vi "NI MAX DAY 2 (11.03.2025) (1).vi"() -> ()   [LabVIEW 2025]
panel:
  out "Boolean 2":bool
  in  "stop 2":bool
  in  "stop":bool
  out "Boolean":bool
  out "Numeric 2":i32
  out "Numeric":i32
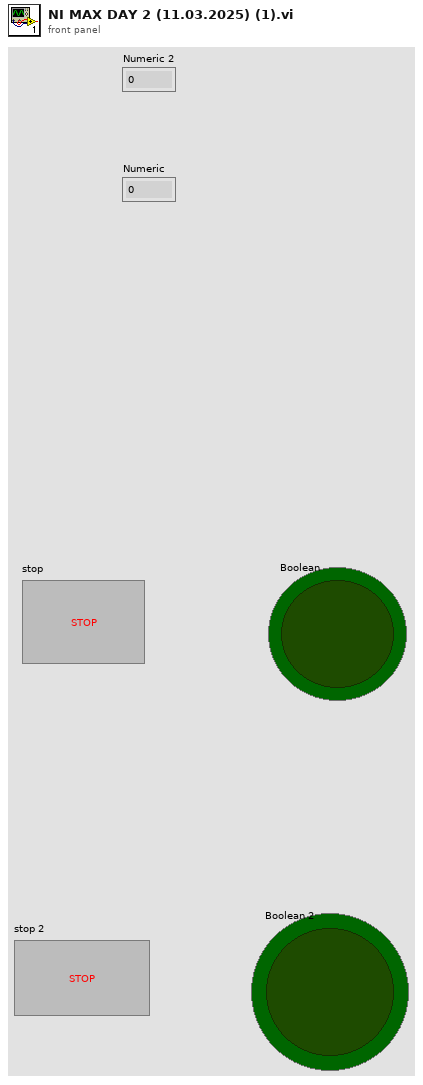
[diagram p1: front panel]
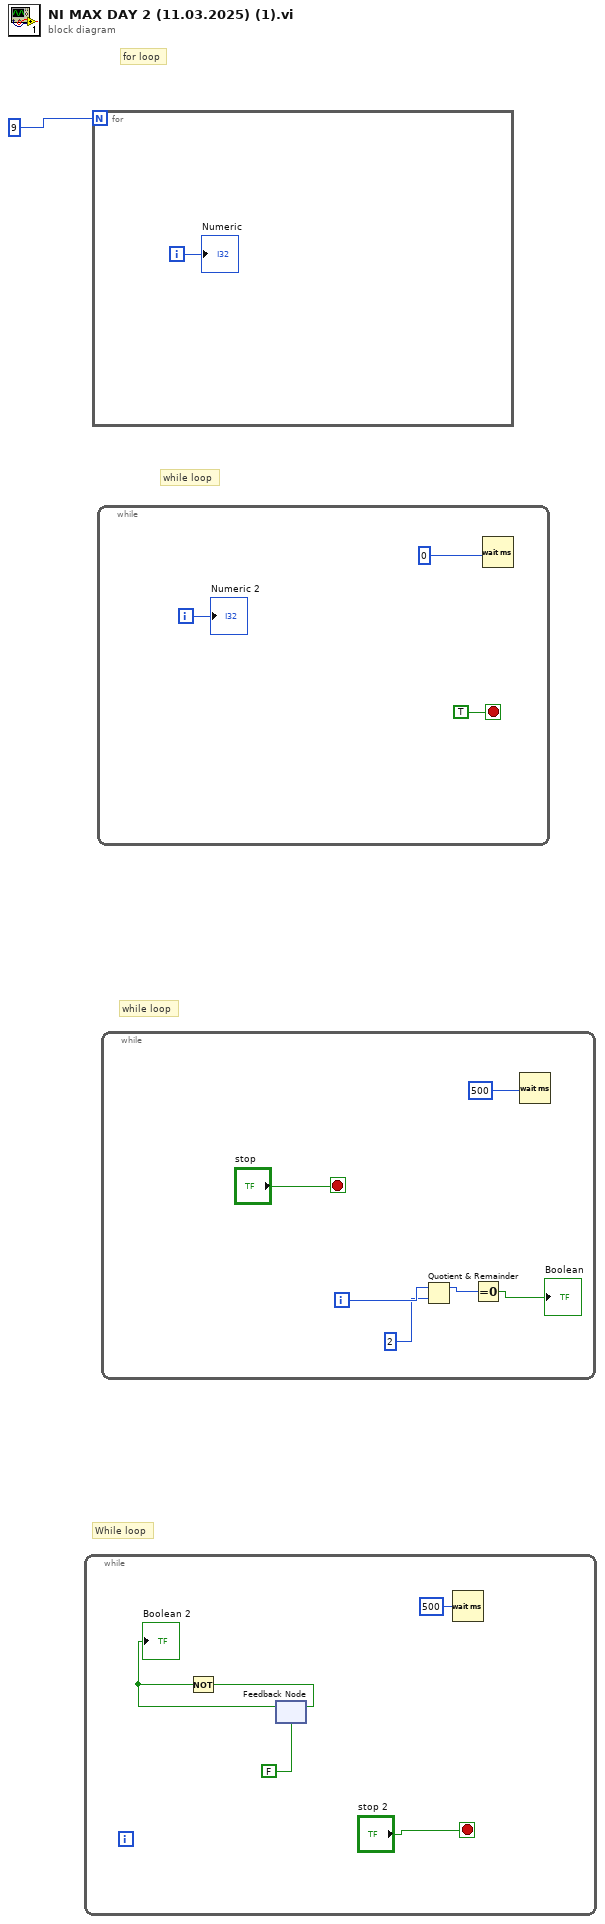
[diagram p0: block diagram]
diagram:
  # "While loop"
  # "for loop"
  # "while loop"
  # "while loop"
  n1 = while {
    stop <- "stop 2" stop-if-true
    n2 = feedback #1(FALSE) -> (w3:bool)
    "Boolean 2" <- w3
    n3 = Not(x=w3) -> (.not. x?=w2:bool)
    n4 = feedback-in #1(w2) -> ()
    n5 = Wait (ms)(milliseconds to wait=u32 500) -> ()  [unwired: 1 out]
  }
  n6 = for {
    N: 9 -> [_]
    i -> [w7]
    "Numeric" <- w7
  }
  n7 = while {
    i -> [w10]
    stop <- TRUE stop-if-true
    n8 = Wait (ms)(milliseconds to wait=u32 0 ("millisecond timer value")) -> ()  [unwired: 1 out]
    "Numeric 2" <- w10
  }
  n9 = while {
    i -> [w14]
    stop <- "stop" stop-if-true
    n10 = Quotient & Remainder(x=w14, y=2 ("floor(x/y)")) -> (x-y*floor(x/y)=w12:i32)  [unwired: 1 out]
    n11 = Equal To 0?(x=w12) -> (x = 0?=→"Boolean":bool)
    n12 = Wait (ms)(milliseconds to wait=u32 500 ("millisecond timer value")) -> ()  [unwired: 1 out]
  }
